vi "Swap.vi"(9 "Y":i32, 10 "X":i32, 11 "Unswapped Array":i32[](array[numeric])) -> (3 "Swapped Array":i32[](array[numeric]))   [LabVIEW 2016]
panel:
  out "Min Index":u32
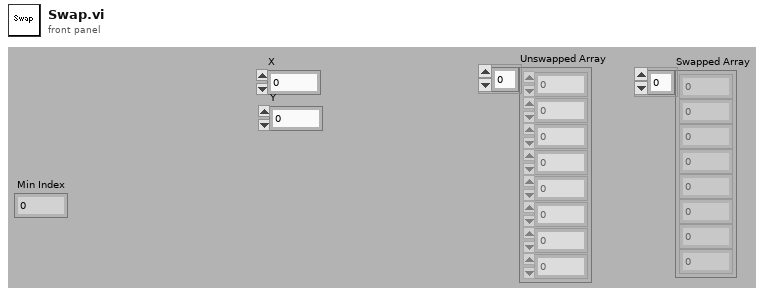
[diagram p1: front panel]
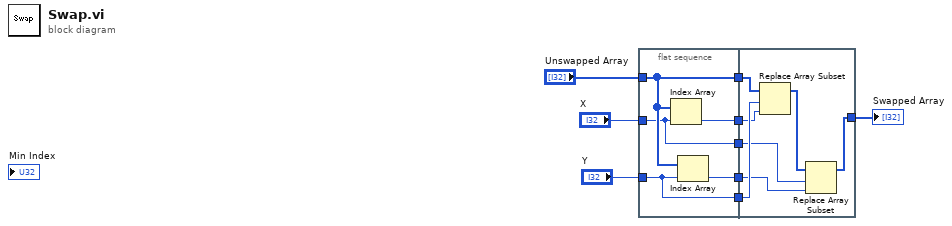
[diagram p0: block diagram]
diagram:
  n1 = flat-sequence {
    tunnel: "Unswapped Array" -> [w11]
    tunnel: [w11] -> w9
    tunnel: "Y" -> [w12]
    tunnel: "X" -> [w10]
    tunnel: [w14] -> w8
    tunnel: [w13] -> w7
    tunnel: [w10] -> w6
    tunnel: [w12] -> w5
    tunnel: w9 -> [w21]
    tunnel: w8 -> [w18]
    tunnel: w7 -> [w16]
    tunnel: w6 -> [w17]
    tunnel: w5 -> [w19]
    tunnel: [w15] -> w1
    frame #0 {
      n2 = Index Array(array=w11, index=w10) -> (element=w14:i32)
      n3 = Index Array(array=w11, index=w12) -> (element=w13:i32)
    }
    frame #1 {
      n4 = Replace Array Subset(array=w21, new element=w18, index=w19) -> (w20:i32[])
      n5 = Replace Array Subset(array=w20, new element=w16, index=w17) -> (w15:i32[])
    }
  }
  "Swapped Array" <- w1
